vi "ARydh -- publish -- handle.vi"(7 "publisher action":T2, 10 "MCL object":T1) -> (2 "MCL object OUT":T1)   [LabVIEW 2019]
uses:
  publisher action.ctl
  Users/Nanocal/Desktop/Calorimetry v1.3/MCL.lvlibp/MCL library/MCL_DataRef.ctl
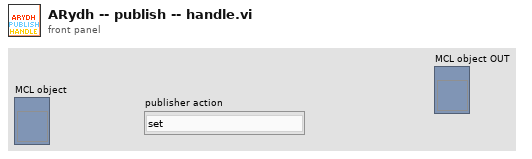
[diagram p1: front panel]
types:
  T1 = typedef "MCL.lvlibp/MCL_DataRef.ctl" = refnum<vi>
  T2 = typedef "publisher action.ctl" = enum16{"set", "get", "init", "check"}
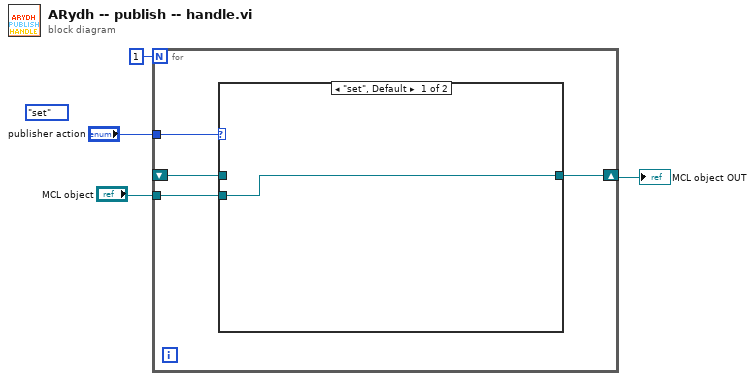
[diagram p0: block diagram]
diagram:
  (unwired) publisher_action."set" ("publisher action")
  n1 = for {
    N: 1 -> [_]
    tunnel: "publisher action" -> [w8]
    tunnel: "MCL object" -> [w6]
    shift-right: [w7] -> w2
    shift-left: _ -> [w5]
    n2 = case shown="\"set\", Default" w8 {
      tunnel: [w9 w10] -> w7
      tunnel: w6 -> [w9 _]
      tunnel: w5 -> [_ w10]
      frame "set", Default {
      }
      frame "get" {
      }
    }
  }
  "MCL object OUT" <- w2
